vi "Coordenadas de obstaculos.vi"(0 "VISA resource name":refnum<visa-resource-name>, 1 "EX2":i32, 2 "EY2":i32, 5 "EX1":i32, 9 "EY1":i32, 11 "error in (no error)":errorcluster, 12 "EX3":i32, 13 "EY3":i32) -> (4 "VISA resource name out":refnum<visa-resource-name>, 15 "error out":errorcluster)   [LabVIEW 2021]
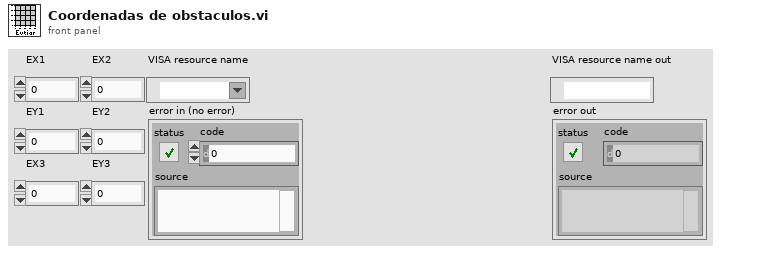
[diagram p1: front panel]
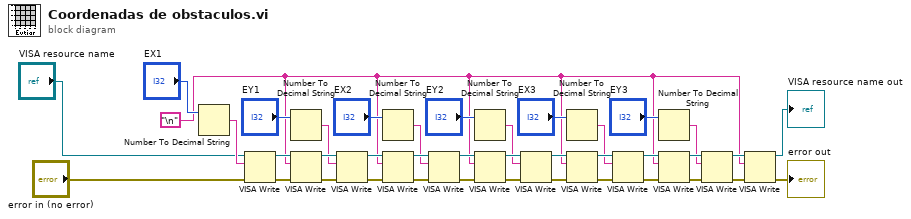
[diagram p0: block diagram]
diagram:
  w3 = "\n"
  n1 = Number To Decimal String(number="EX1") -> (decimal integer string=w30:string)  [unwired: 1 in]
  n2 = VISA Write(VISA resource name="VISA resource name", write buffer=w30, error in (no error)="error in (no error)") -> (VISA resource name out=w38:refnum<visa-resource-name>, error out=w39:errorcluster)  [unwired: 1 out]
  n3 = Number To Decimal String(number="EY1") -> (decimal integer string=w29:string)  [unwired: 1 in]
  n4 = VISA Write(VISA resource name=w38, write buffer=w3, error in (no error)=w39) -> (VISA resource name out=w37:refnum<visa-resource-name>, error out=w36:errorcluster)  [unwired: 1 out]
  n5 = VISA Write(VISA resource name=w37, write buffer=w29, error in (no error)=w36) -> (VISA resource name out=w35:refnum<visa-resource-name>, error out=w34:errorcluster)  [unwired: 1 out]
  n6 = Number To Decimal String(number="EX2") -> (decimal integer string=w19:string)  [unwired: 1 in]
  n7 = VISA Write(VISA resource name=w35, write buffer=w3, error in (no error)=w34) -> (VISA resource name out=w27:refnum<visa-resource-name>, error out=w28:errorcluster)  [unwired: 1 out]
  n8 = VISA Write(VISA resource name=w27, write buffer=w19, error in (no error)=w28) -> (VISA resource name out=w25:refnum<visa-resource-name>, error out=w26:errorcluster)  [unwired: 1 out]
  n9 = Number To Decimal String(number="EY2") -> (decimal integer string=w18:string)  [unwired: 1 in]
  n10 = VISA Write(VISA resource name=w25, write buffer=w3, error in (no error)=w26) -> (VISA resource name out=w23:refnum<visa-resource-name>, error out=w24:errorcluster)  [unwired: 1 out]
  n11 = VISA Write(VISA resource name=w23, write buffer=w18, error in (no error)=w24) -> (VISA resource name out=w21:refnum<visa-resource-name>, error out=w22:errorcluster)  [unwired: 1 out]
  n12 = Number To Decimal String(number="EX3") -> (decimal integer string=w8:string)  [unwired: 1 in]
  n13 = VISA Write(VISA resource name=w21, write buffer=w3, error in (no error)=w22) -> (VISA resource name out=w16:refnum<visa-resource-name>, error out=w17:errorcluster)  [unwired: 1 out]
  n14 = VISA Write(VISA resource name=w16, write buffer=w8, error in (no error)=w17) -> (VISA resource name out=w14:refnum<visa-resource-name>, error out=w15:errorcluster)  [unwired: 1 out]
  n15 = Number To Decimal String(number="EY3") -> (decimal integer string=w6:string)  [unwired: 1 in]
  n16 = VISA Write(VISA resource name=w14, write buffer=w3, error in (no error)=w15) -> (VISA resource name out=w12:refnum<visa-resource-name>, error out=w13:errorcluster)  [unwired: 1 out]
  n17 = VISA Write(VISA resource name=w12, write buffer=w6, error in (no error)=w13) -> (VISA resource name out=w10:refnum<visa-resource-name>, error out=w11:errorcluster)  [unwired: 1 out]
  n18 = VISA Write(VISA resource name=w10, write buffer=w3, error in (no error)=w11) -> (VISA resource name out=→"VISA resource name out":refnum<visa-resource-name>, error out=→"error out":errorcluster)  [unwired: 1 out]
